vi "Set Theme Data.vi"(7 "VI Refnum":refnum<vi>, 8 "error in":errorcluster, 10 "Theme":u16(ring)=3 items=["Light Theme", "Light Medium Contrast", "Light High Contrast", "Dark Theme", "Dark Medium Contrast", "Dark High Constrast"], 11 "Material Theme.lvclass":refnum<class "Material Theme.lvclass">) -> (0 "error out":errorcluster)   [LabVIEW 2021, in "TSC Material Theme.lvlib" / "Material Theme.lvclass"]
doc: "Set the VI's User Tag data to track the theme and theme mode applied.\n\n<b>Code Developed By:</b>\nDaniel Coons\nTechnology Service Corporation\nwww.tsc.com/atcs"
uses:
  Material Theme.lvclass
  Material Theme.lvclass/Material Theme.ctl
  <vilib>/UserTags/UserTags.lvlib
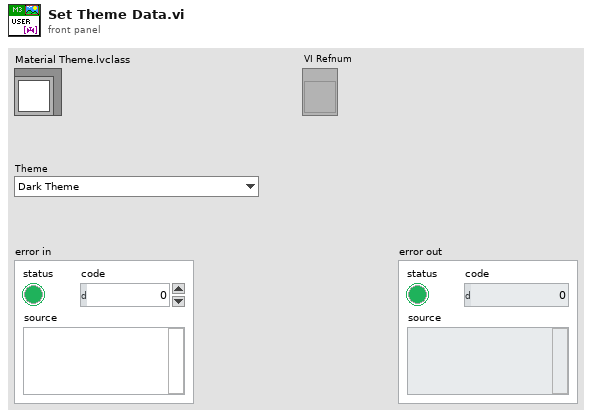
[diagram p1: front panel]
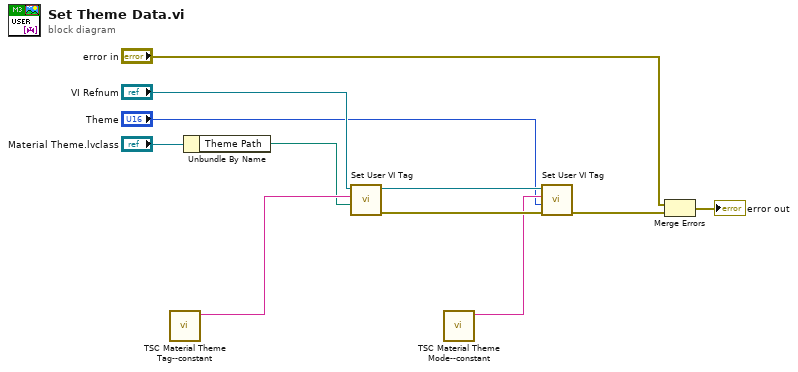
[diagram p0: block diagram]
diagram:
  n1 = call "TSC Material Theme Tag--constant.vi"() -> ("Theme Path Tag"=w7:string)  [unwired: 11 in]
  n2 = Unbundle By Name("Material Theme.lvclass") -> ("Theme Path"=w5:path)
  n3 = call <vilib>:"Set User VI Tag.vi"("Value"=w5, "Tag Name"=w7, "VI Refnum"="VI Refnum") -> ("error out"=w11:errorcluster, "dup VI Refnum"=w8:refnum<vi>)  [unwired: 6 in, 1 out]
  n4 = call "TSC Material Theme Mode--constant.vi"() -> ("Theme Path Tag"=w4:string)  [unwired: 11 in]
  n5 = call <vilib>:"Set User VI Tag.vi"("error in (no error)"=w11, "Value"="Theme", "Tag Name"=w4, "VI Refnum"=w8) -> ("error out"=w10:errorcluster)  [unwired: 5 in, 2 out]
  n6 = Merge Errors("error in", w10) -> (→"error out":errorcluster)
